vi "DCPower_CurrentLimitConfiguration.vi"(8 "error in (no error)":errorcluster, 9 "current limit":dbl, 10 "Active Channel Numbers String":string, 11 "IVI Refnum in":refnum<k15>) -> (0 "error out":errorcluster, 3 "IVI Refnum out":refnum<k15>)   [LabVIEW 2019]
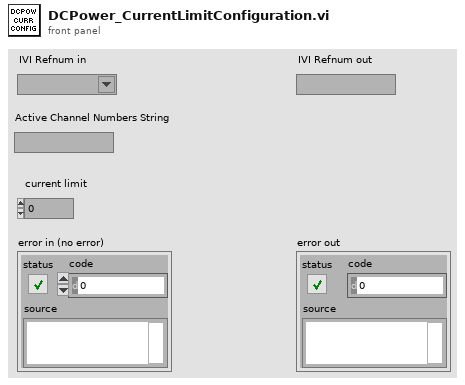
[diagram p1: front panel]
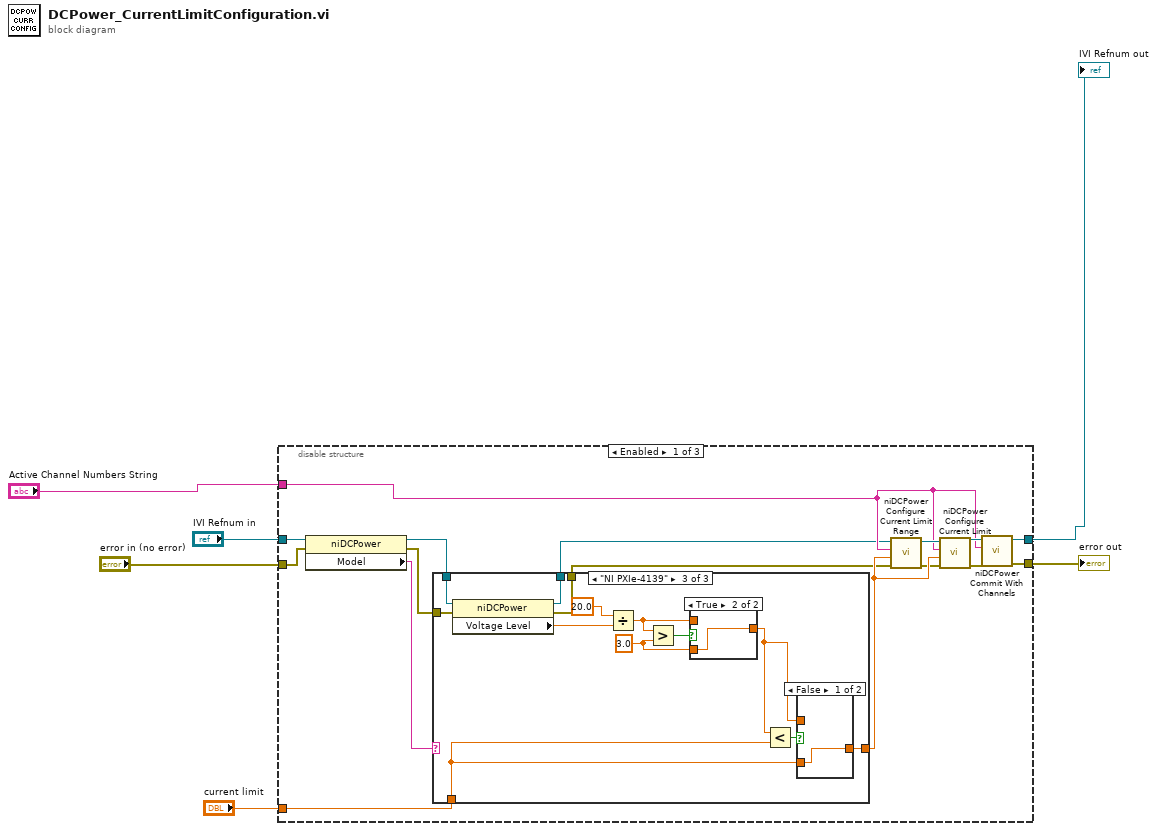
[diagram p0: block diagram]
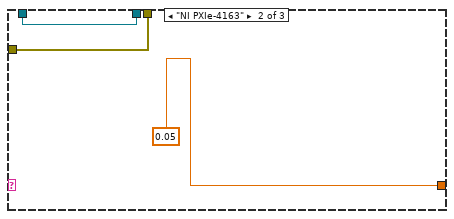
[diagram p3: hidden frame]
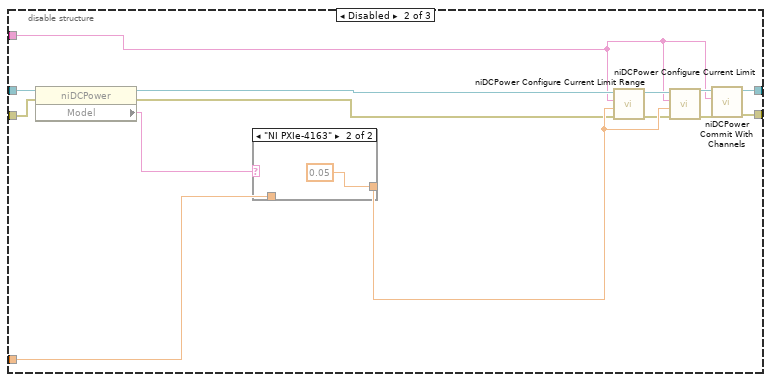
[diagram p6: hidden frame]
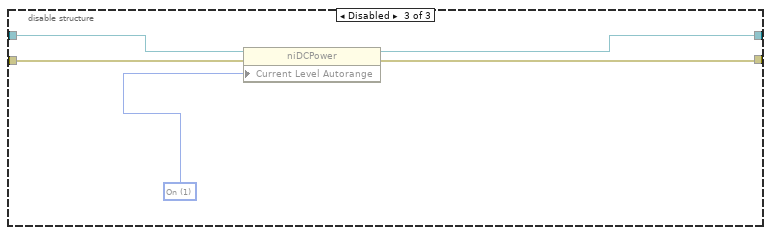
[diagram p8: hidden frame]
diagram:
  n1 = disable-structure shown="Enabled" {
    disable-tunnel: [w22 w59 w62] -> w6
    disable-tunnel: [w21 w58 w63] -> w5
    disable-tunnel: "current limit" -> [w20 w57 _]
    disable-tunnel: "error in (no error)" -> [w19 w56 w64]
    disable-tunnel: "IVI Refnum in" -> [w18 w55 w65]
    disable-tunnel: "Active Channel Numbers String" -> [w11 w46 _]
    frame Enabled {
      n2 = property class="niDCPower"(reference=w18, error in=w19) -> (reference out=w9:refnum<k15>, error out=w10:errorcluster, "Model"=w14:string)
      n3 = case shown="\"NI PXIe-4139\"" w14 {
        tunnel: w20 -> [w25 _ w36]
        tunnel: [w25 0.05 ("current limit") w34] -> w15
        tunnel: w10 -> [w23 w27 w32]
        tunnel: w9 -> [w24 w26 w31]
        tunnel: [w23 w27 w29] -> w7
        tunnel: [w24 w26 w30] -> w8
        frame Default {
        }
        frame "NI PXIe-4163" {
        }
        frame "NI PXIe-4139" {
          w38 = 3.0 ("y")
          n4 = property class="niDCPower"(reference=w31, error in=w32) -> (reference out=w30:refnum<k15>, error out=w29:errorcluster, "Voltage Level"=w33:dbl)
          n5 = Divide(x=20.0, y=w33) -> (x/y=w39:dbl)
          n6 = Greater?(x=w39, y=w38) -> (0:w40:bool)
          n7 = case shown="True" w40 {
            tunnel: [w44 w45] -> w35
            tunnel: w39 -> [w44 _]
            tunnel: w38 -> [_ w45]
            frame False {
            }
            frame True {
            }
          }
          n8 = Less?(x=w35, y=w36) -> (x < y?=w37:bool)
          n9 = case shown="False" w37 {
            tunnel: w35 -> [_ w43]
            tunnel: w36 -> [w42 _]
            tunnel: [w42 w43] -> w34
            frame False {
            }
            frame True {
            }
          }
        }
      }
      n10 = call <instrlib>:"niDCPower Configure Current Limit Range.vi"("error in (no error)"=w7, "current limit range"=w15, "channel name"=w11, "instrument handle"=w8) -> ("error out"=w12:errorcluster, "instrument handle out"=w13:refnum<k15>)  [unwired: 6 in]
      n11 = call <instrlib>:"niDCPower Configure Current Limit.vi"("error in (no error)"=w12, "current limit"=w15, "channel name"=w11, "instrument handle"=w13) -> ("error out"=w17:errorcluster, "instrument handle out"=w16:refnum<k15>)  [unwired: 6 in]
      n12 = call <instrlib>:"niDCPower Commit With Channels.vi"("error in (no error)"=w17, "channel name"=w11, "instrument handle"=w16) -> ("error out"=w22:errorcluster, "instrument handle out"=w21:refnum<k15>)  [unwired: 7 in]
    }
    frame Disabled {
      n13 = property class="niDCPower"(reference=w55, error in=w56) -> (reference out=w49:refnum<k15>, error out=w50:errorcluster, "Model"=w51:string)
      n14 = case shown="\"NI PXIe-4163\"" w51 {
        tunnel: w57 -> [w60 _]
        tunnel: [w60 0.05 ("current limit")] -> w52
        frame Default {
        }
        frame "NI PXIe-4163" {
        }
      }
      n15 = call <instrlib>:"niDCPower Configure Current Limit Range.vi"("error in (no error)"=w50, "current limit range"=w52, "channel name"=w46, "instrument handle"=w49) -> ("error out"=w47:errorcluster, "instrument handle out"=w48:refnum<k15>)  [unwired: 6 in]
      n16 = call <instrlib>:"niDCPower Configure Current Limit.vi"("error in (no error)"=w47, "current limit"=w52, "channel name"=w46, "instrument handle"=w48) -> ("error out"=w54:errorcluster, "instrument handle out"=w53:refnum<k15>)  [unwired: 6 in]
      n17 = call <instrlib>:"niDCPower Commit With Channels.vi"("error in (no error)"=w54, "channel name"=w46, "instrument handle"=w53) -> ("error out"=w59:errorcluster, "instrument handle out"=w58:refnum<k15>)  [unwired: 7 in]
    }
    frame Disabled {
      w66 = 1 items=["Off", "On"] ("Source:DC Current:Current Level Autorange")
      n18 = property class="niDCPower"(reference=w65, error in=w64, "Current Level Autorange"=w66) -> (reference out=w63:refnum<k15>, error out=w62:errorcluster)
    }
  }
  "error out" <- w6
  "IVI Refnum out" <- w5
